vi "Call Core.vi"(8 "error in (no error)":errorcluster, 11 "Scenarios Class in":refnum<class "Scenarios Class.lvclass">) -> (0 "error out":errorcluster, 3 "Scenarios Class out":refnum<class "Scenarios Class.lvclass">)   [LabVIEW 2020, in "SECS Scenarios.lvlib" / "Scenarios Class.lvclass"]
uses:
  Scenarios Class.lvclass
  Core.vi
  Scenarios Class.lvclass/Scenarios Class.ctl
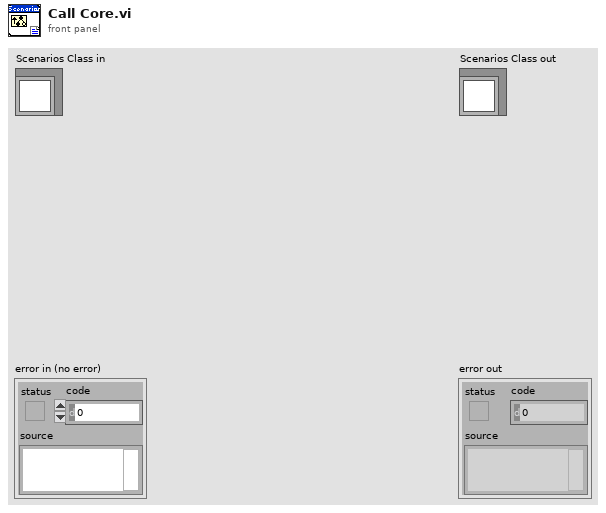
[diagram p1: front panel]
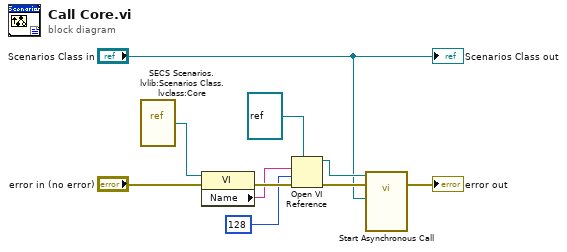
[diagram p0: block diagram]
diagram:
  n1 = vi-ref "SECS Scenarios.lvlib:Scenarios Class.lvclass:Core.vi"() -> (w9:refnum<vi>)
  n2 = property class="VI"(reference=w9, error in="error in (no error)") -> (error out=w8:errorcluster, "Name"=w7:string)  [unwired: 1 out]
  n3 = Open VI Reference(type specifier VI Refnum (for type only)=refnum<vi> refnum, vi path=w7, options=128, error in (no error)=w8) -> (vi reference=w3:refnum<vi>, error out=w4:errorcluster)  [unwired: 2 in]
  n4 = call-by-ref "Start Asynchronous Call"(reference=w3, error in=w4, "Scenarios Class in"="Scenarios Class in") -> (error out=→"error out":errorcluster)  [unwired: 9 in, 3 out]
  "Scenarios Class out" <- "Scenarios Class in"
